vi "Cal ColNum(SubVI) - rgb.vi"(6 "Ready For Input":bool, 8 "DV":bool, 10 "Width":u16, 11 "preCol":u16) -> (2 "curCol":u16)   [LabVIEW 2016]
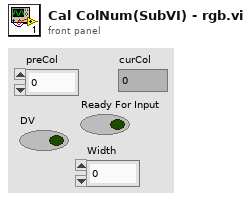
[diagram p1: front panel]
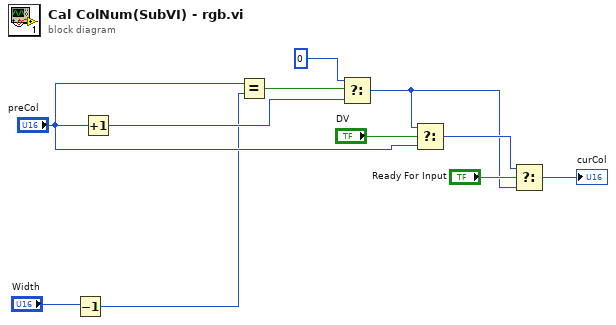
[diagram p0: block diagram]
diagram:
  n1 = Decrement(x="Width") -> (x-1=w2:u16)
  n2 = Increment(x="preCol") -> (x+1=w4:u16)
  n3 = Equal?(x="preCol", y=w2) -> (x = y?=w6:bool)
  n4 = Select(t=i16 0, s=w6, f=w4) -> (s? t:f=w1:u16)
  n5 = Select(t=w1, s="DV", f="preCol") -> (s? t:f=w9:u16)
  n6 = Select(t=w9, s="Ready For Input", f=w1) -> (s? t:f=→"curCol":u16)
